vi "Get BuildWorker Name.vi"(8 "error in (no error)":errorcluster, 11 "BuildWorker Basics in":refnum<class "BuildWorker Local.lvclass">) -> (0 "error out":errorcluster, 2 "Name":string, 3 "BuildWorker Basics out":refnum<class "BuildWorker Local.lvclass">)   [LabVIEW 2017, in "BuildWorker Interface.lvlib" / "BuildWorker Local.lvclass"]
uses:
  BuildWorker Local.lvclass
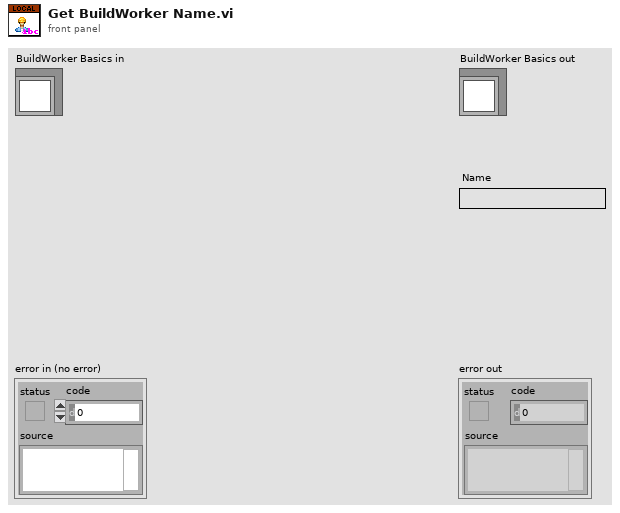
[diagram p1: front panel]
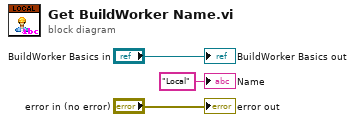
[diagram p0: block diagram]
diagram:
  "error out" <- "error in (no error)"
  "BuildWorker Basics out" <- "BuildWorker Basics in"
  "Name" <- "Local" ("Name")
